vi "Write Square Esitmated Sum.vi"(8 "error in (no error)":errorcluster, 10 "Square Esitmated Sum":dbl, 11 "Online_TRAC in":refnum<class "Online_TRAC.lvclass">) -> (0 "error out":errorcluster, 3 "Online_TRAC out":refnum<class "Online_TRAC.lvclass">)   [LabVIEW 2021, in "Online_TRAC.lvclass"]
uses:
  Online_TRAC.lvclass
  Online_TRAC.lvclass/Online_TRAC.ctl
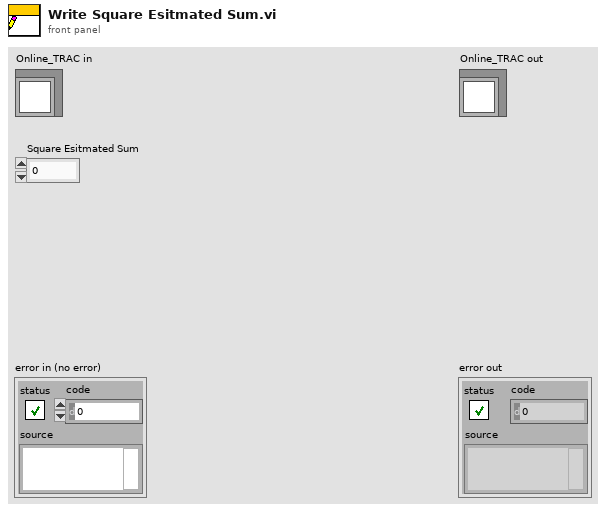
[diagram p1: front panel]
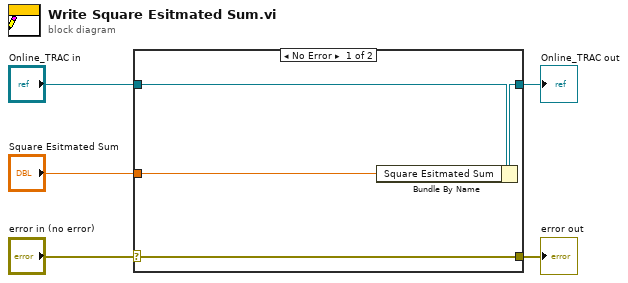
[diagram p0: block diagram]
diagram:
  n1 = case shown="No Error" "error in (no error)" {
    selector: "error in (no error)" -> [w9 w10]
    tunnel: [w9 w10] -> w4
    tunnel: [w7 w11] -> w2
    tunnel: "Online_TRAC in" -> [w8 w11]
    tunnel: "Square Esitmated Sum" -> [w6 _]
    frame No Error {
      n2 = Bundle By Name(cluster=w8, "Square Esitmated Sum"=w6) -> (w7:refnum<class "Online_TRAC.lvclass">)
    }
    frame Error {
    }
  }
  "error out" <- w4
  "Online_TRAC out" <- w2
